vi "GEOM_BinCoords.vi"(10 "Binning":T2={"x"=1, "y"=1} {"y" min=1; "x" min=1}, 11 "coords":T1={"xstart"=1, "ystart"=1, "xsize"=1, "ysize"=1}) -> (1 "remaining Y":i32, 2 "remainingX":i32, 3 "binnedcoords":T1={"xstart"=1, "ystart"=1, "xsize"=1, "ysize"=1})   [LabVIEW 2016]
uses:
  GEOM_Binning.ctl
  GEOM_Coords.ctl
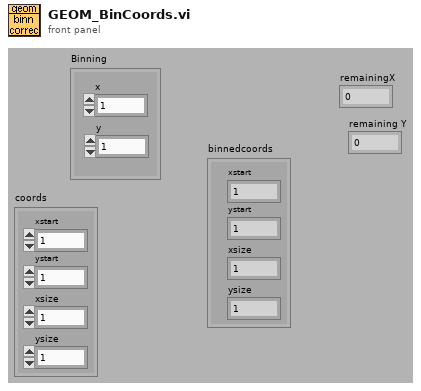
[diagram p1: front panel]
types:
  T1 = typedef "GEOM_Coords.ctl" = cluster{"xstart":u32, "ystart":u32, "xsize":u32, "ysize":u32}
  T2 = typedef "GEOM_Binning.ctl" = cluster{"x":u32, "y":u32}
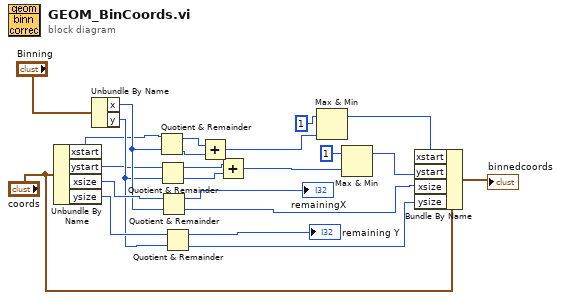
[diagram p0: block diagram]
diagram:
  n1 = Unbundle By Name("coords") -> ("xstart"=w5:u32, "ystart"=w4:u32, "xsize"=w20:u32, "ysize"=w19:u32)
  n2 = Unbundle By Name("Binning") -> ("x"=w18:u32, "y"=w17:u32)
  n3 = Quotient & Remainder(x=w5, y=w18) -> (x-y*floor(x/y)=w7:u32, floor(x/y)=w8:u32)
  n4 = Quotient & Remainder(x=w4, y=w17) -> (x-y*floor(x/y)=w3:u32, floor(x/y)=w1:u32)
  n5 = Quotient & Remainder(x=w20, y=w18) -> (x-y*floor(x/y)=→"remainingX":u32, floor(x/y)=w16:u32)
  n6 = Quotient & Remainder(x=w19, y=w17) -> (x-y*floor(x/y)=→"remaining Y":u32, floor(x/y)=w15:u32)
  n7 = Add(x=w7, y=w8) -> (x+y=w6:u32)
  n8 = Add(x=w3, y=w1) -> (x+y=w2:u32)
  n9 = Max & Min(x=u32 1, y=w6) -> (max(x,y)=w11:u32)  [unwired: 1 out]
  n10 = Max & Min(x=u32 1, y=w2) -> (max(x,y)=w9:u32)  [unwired: 1 out]
  n11 = Bundle By Name(cluster="coords", "xstart"=w11, "ystart"=w9, "xsize"=w16, "ysize"=w15) -> (→"binnedcoords":T1)
